vi "Keithley 622x Set Delta.vi"(4 "Max readings":string="INF", 6 "Step":dbl=0.0001 format="%#_6p", 7 "Delta":dbl=0.0001 format="%#_6p", 8 "error in":errorcluster, 9 "End":dbl=0.001 format="%#_6p", 10 "Start":dbl=-0.001 format="%#_6p", 11 "VISA resource name":refnum<visa-resource-name>) -> (0 "error out":errorcluster, 3 "VISA resource name out":refnum<visa-resource-name>)   [LabVIEW 2021]
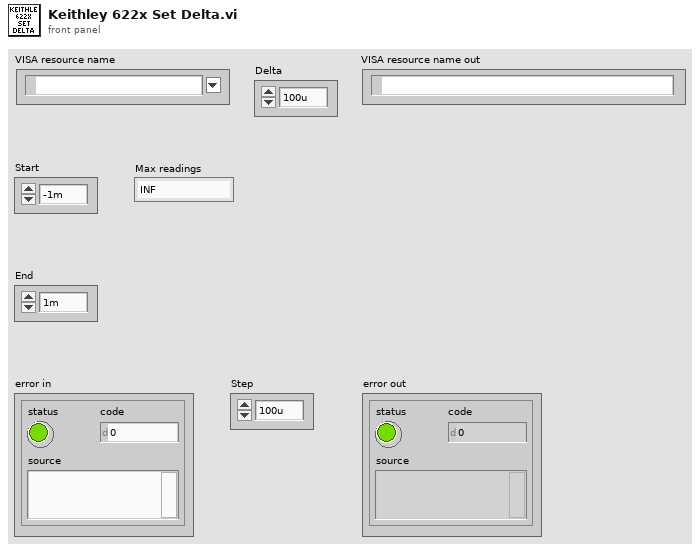
[diagram p1: front panel]
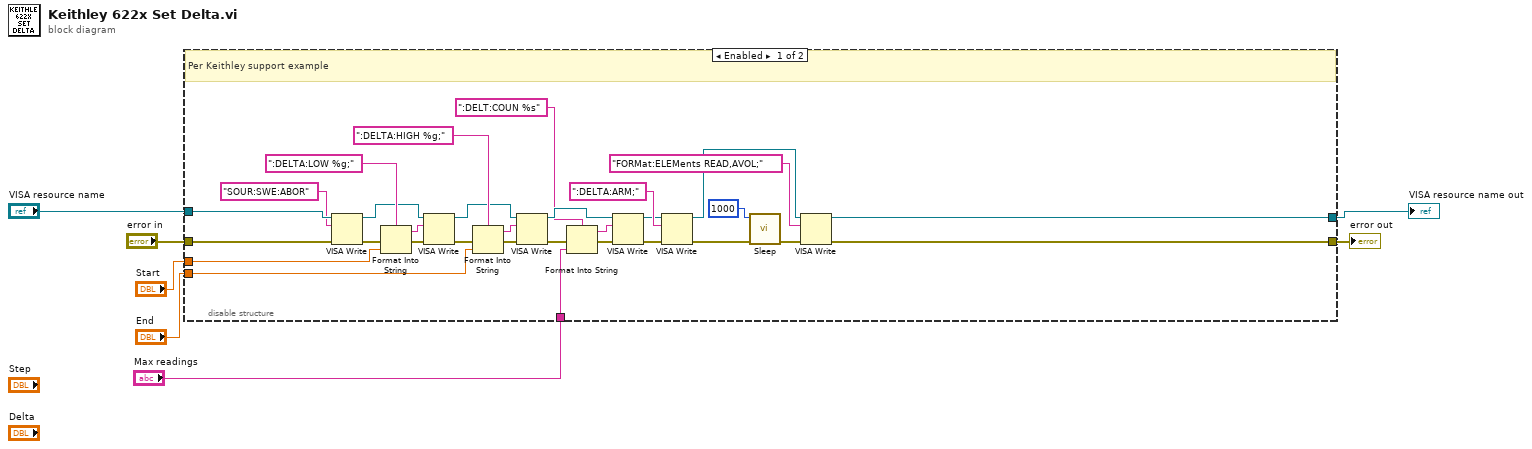
[diagram p0: block diagram]
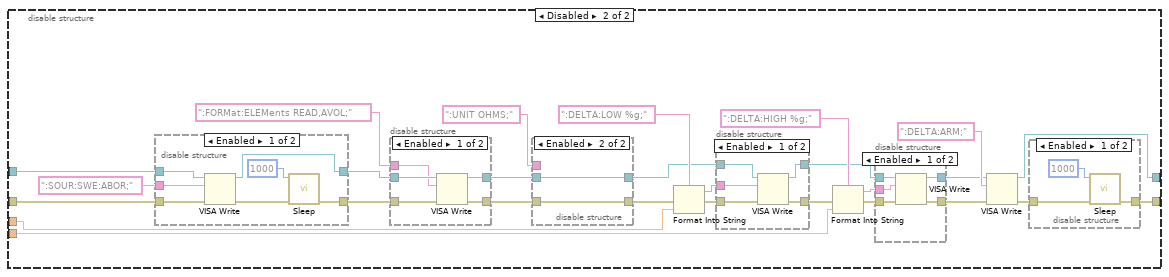
[diagram p2: hidden frame]
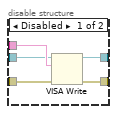
[diagram p6: hidden frame]
diagram:
  n1 = disable-structure shown="Enabled" {
    disable-tunnel: "Start" -> [w36 w62]
    disable-tunnel: [w13 w59] -> w6
    disable-tunnel: [w15 w58] -> w5
    disable-tunnel: "End" -> [w30 w54]
    disable-tunnel: "VISA resource name" -> [w24 w44]
    disable-tunnel: "error in" -> [w23 w43]
    disable-tunnel: "Max readings" -> [w8 _]
    frame Enabled {
      # "Per Keithley support example"
      n2 = VISA Write(VISA resource name=w24, write buffer="SOUR:SWE:ABOR", error in (no error)=w23) -> (VISA resource name out=w26:refnum<visa-resource-name>, error out=w25:errorcluster)  [unwired: 1 out]
      n3 = Format Into String(format string=":DELTA:LOW %g;", error in=w25, w36) -> (resulting string=w37:string, error out=w38:errorcluster)  [unwired: 1 in]
      n4 = VISA Write(VISA resource name=w26, write buffer=w37, error in (no error)=w38) -> (VISA resource name out=w28:refnum<visa-resource-name>, error out=w27:errorcluster)  [unwired: 1 out]
      n5 = Format Into String(format string=":DELTA:HIGH %g;", error in=w27, w30) -> (resulting string=w32:string, error out=w31:errorcluster)  [unwired: 1 in]
      n6 = VISA Write(VISA resource name=w28, write buffer=w32, error in (no error)=w31) -> (VISA resource name out=w19:refnum<visa-resource-name>, error out=w12:errorcluster)  [unwired: 1 out]
      n7 = Format Into String(format string=":DELT:COUN %s", error in=w12, w8) -> (resulting string=w9:string, error out=w11:errorcluster)  [unwired: 1 in]
      n8 = VISA Write(VISA resource name=w19, write buffer=w9, error in (no error)=w11) -> (VISA resource name out=w18:refnum<visa-resource-name>, error out=w20:errorcluster)  [unwired: 1 out]
      n9 = VISA Write(VISA resource name=w18, write buffer=":DELTA:ARM;", error in (no error)=w20) -> (VISA resource name out=w14:refnum<visa-resource-name>, error out=w35:errorcluster)  [unwired: 1 out]
      n10 = call "Sleep.vi"("error in"=w35, "milliseconds to wait"=u32 1000) -> ("error out"=w17:errorcluster)  [unwired: 9 in]
      n11 = VISA Write(VISA resource name=w14, write buffer="FORMat:ELEMents READ,AVOL;", error in (no error)=w17) -> (VISA resource name out=w13:refnum<visa-resource-name>, error out=w15:errorcluster)  [unwired: 1 out]
    }
    frame Disabled {
      n12 = disable-structure shown="Enabled" {
        disable-tunnel: [w80 w87] -> w42
        disable-tunnel: ":SOUR:SWE:ABOR;" -> [w86 _]
        disable-tunnel: [w85 w88] -> w41
        disable-tunnel: w44 -> [w84 w88]
        disable-tunnel: w43 -> [w83 w87]
        frame Enabled {
          n13 = VISA Write(VISA resource name=w84, write buffer=w86, error in (no error)=w83) -> (VISA resource name out=w85:refnum<visa-resource-name>, error out=w81:errorcluster)  [unwired: 1 out]
          n14 = call "Sleep.vi"("error in"=w81, "milliseconds to wait"=u32 1000) -> ("error out"=w80:errorcluster)  [unwired: 9 in]
        }
        frame Disabled {
        }
      }
      n15 = disable-structure shown="Enabled" {
        disable-tunnel: w41 -> [w100 w102]
        disable-tunnel: ":FORMat:ELEMents READ,AVOL;" -> [w99 _]
        disable-tunnel: w42 -> [w98 w101]
        disable-tunnel: [w97 w101] -> w45
        disable-tunnel: [w96 w102] -> w46
        frame Enabled {
          n16 = VISA Write(VISA resource name=w100, write buffer=w99, error in (no error)=w98) -> (VISA resource name out=w96:refnum<visa-resource-name>, error out=w97:errorcluster)  [unwired: 1 out]
        }
        frame Disabled {
        }
      }
      n17 = disable-structure shown="Enabled" {
        disable-tunnel: ":UNIT OHMS;" -> [w93 _]
        disable-tunnel: [w92 w95] -> w39
        disable-tunnel: w46 -> [w91 w95]
        disable-tunnel: w45 -> [w90 w94]
        disable-tunnel: [w89 w94] -> w40
        frame Disabled {
          n18 = VISA Write(VISA resource name=w91, write buffer=w93, error in (no error)=w90) -> (VISA resource name out=w92:refnum<visa-resource-name>, error out=w89:errorcluster)  [unwired: 1 out]
        }
        frame Enabled {
        }
      }
      n19 = Format Into String(format string=":DELTA:LOW %g;", error in=w40, w62) -> (resulting string=w64:string, error out=w65:errorcluster)  [unwired: 1 in]
      n20 = disable-structure shown="Enabled" {
        disable-tunnel: w65 -> [w70 w71]
        disable-tunnel: w64 -> [w69 _]
        disable-tunnel: [w68 w72] -> w52
        disable-tunnel: [w67 w71] -> w50
        disable-tunnel: w39 -> [w66 w72]
        frame Enabled {
          n21 = VISA Write(VISA resource name=w66, write buffer=w69, error in (no error)=w70) -> (VISA resource name out=w68:refnum<visa-resource-name>, error out=w67:errorcluster)  [unwired: 1 out]
        }
        frame Disabled {
        }
      }
      n22 = Format Into String(format string=":DELTA:HIGH %g;", error in=w50, w54) -> (resulting string=w56:string, error out=w55:errorcluster)  [unwired: 1 in]
      n23 = disable-structure shown="Enabled" {
        disable-tunnel: w56 -> [w77 _]
        disable-tunnel: w55 -> [w76 w78]
        disable-tunnel: w52 -> [w75 w79]
        disable-tunnel: [w74 w79] -> w51
        disable-tunnel: [w73 w78] -> w49
        frame Enabled {
          n24 = VISA Write(VISA resource name=w75, write buffer=w77, error in (no error)=w76) -> (VISA resource name out=w74:refnum<visa-resource-name>, error out=w73:errorcluster)  [unwired: 1 out]
        }
        frame Disabled {
        }
      }
      n25 = VISA Write(VISA resource name=w51, write buffer=":DELTA:ARM;", error in (no error)=w49) -> (VISA resource name out=w59:refnum<visa-resource-name>, error out=w61:errorcluster)  [unwired: 1 out]
      n26 = disable-structure shown="Enabled" {
        disable-tunnel: [w105 w106] -> w58
        disable-tunnel: w61 -> [w103 w106]
        frame Enabled {
          n27 = call "Sleep.vi"("error in"=w103, "milliseconds to wait"=u32 1000) -> ("error out"=w105:errorcluster)  [unwired: 9 in]
        }
        frame Disabled {
        }
      }
    }
  }
  "VISA resource name out" <- w6
  "error out" <- w5
